vi "AutoSpotting.vi"(3 "spotfinding settings":T1={"show all"=FALSE, "threshold/morph"=FALSE, "particle filter"=FALSE, "spot marks"=FALSE, "close filter"=FALSE, "connectivity 4/8"=FALSE, "range"={"Lower value"=30.0, "Upper value"=30.0}, "PSF-size"=0, "Parameters"=[]} {"range"."Upper value" format="%.2f"; "range"."Lower value" format="%.2f"; "Parameters"."Upper Value" format="%.2f"; "Parameters"."Lower Value" format="%.2f"}, 4 "Intensity Image In":T2, 5 "already x spots":i16) -> (0 "coordinates":i32[][](array[numeric]), 1 "Number of Particles":i32)   [LabVIEW 2009]
uses:
  <vilib>/vision/Image Controls.llb/IMAQ Image.ctl
  spotfindersettings.ctl
  <vilib>/vision/NI_Vision_Development_Module.lvlib
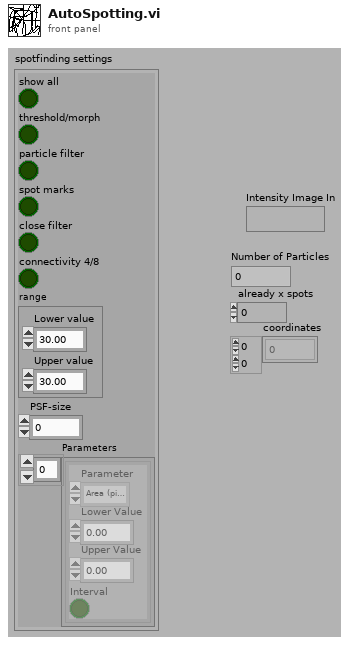
[diagram p1: front panel]
types:
  T1 = typedef "spotfindersettings.ctl" = cluster{"show all":bool, "threshold/morph":bool, "particle filter":bool, "spot marks":bool, "close filter":bool, "connectivity 4/8":bool, "range":cluster{"Lower value":sgl, "Upper value":sgl}, "PSF-size":i32, "Parameters":cluster{"Parameter":enum32{"Area (pixels)", "Area (calibrated)", "Number of holes", "Holes area (pixels)", "Total area (pixels)", "Scanned area (pixels)", "Ratio Area/Scanned area (%)", "Ratio Area/Total area (%)", "Center of mass (X)", "Center of mass (Y)", "Left column (X)", "Upper row (Y)", "Right column (X)", "Lower row (Y)", "Width (pixels)", "Height (pixels)", "Longest segment length", "Longest segment left column (X)", "Longest segment top row  (Y)", "Perimeter", "Holes perimeter", "SumX", "SumY", "SumXX", "SumYY", "SumXY", "Corrected projection X", "Corrected projection Y", "Moment of inertia Ixx", "Moment of inertia Iyy", "Moment of inertia Ixy", "Mean chord X", "Mean chord Y", "Max intercept", "Mean intercept perpendicular", "Particle orientation", "Equivalent ellipse minor axis", "Ellipse major axis", "Ellipse minor axis", "Ratio of equivalent ellipse axis", "Rectangle big side", "Rectangle small side", "Ratio of equivalent rectangle sides", "Elongation factor", "Compactness factor", "Heywood circularity factor", "Type factor", "Hydraulic radius", "Waddel disk diameter", "Diagonal"}, "Lower Value":sgl, "Upper Value":sgl, "Interval":bool}[]}
  T2 = typedef "IMAQ Image.ctl" = refnum<image>
  T3 = enum16{"Ini", "Get", "Set", "Refresh", "dump", "move", "name"}
  T4 = cluster{"Parameter":enum32{"Area (pixels)", "Area (calibrated)", "Number of holes", "Holes area (pixels)", "Total area (pixels)", "Scanned area (pixels)", "Ratio Area/Scanned area (%)", "Ratio Area/Total area (%)", "Center of mass (X)", "Center of mass (Y)", "Left column (X)", "Upper row (Y)", "Right column (X)", "Lower row (Y)", "Width (pixels)", "Height (pixels)", "Longest segment length", "Longest segment left column (X)", "Longest segment top row  (Y)", "Perimeter", "Holes perimeter", "SumX", "SumY", "SumXX", "SumYY", "SumXY", "Corrected projection X", "Corrected projection Y", "Moment of inertia Ixx", "Moment of inertia Iyy", "Moment of inertia Ixy", "Mean chord X", "Mean chord Y", "Max intercept", "Mean intercept perpendicular", "Particle orientation", "Equivalent ellipse minor axis", "Ellipse major axis", "Ellipse minor axis", "Ratio of equivalent ellipse axis", "Rectangle big side", "Rectangle small side", "Ratio of equivalent rectangle sides", "Elongation factor", "Compactness factor", "Heywood circularity factor", "Type factor", "Hydraulic radius", "Waddel disk diameter", "Diagonal"}, "Lower Value":sgl, "Upper Value":sgl, "Interval":bool}[]
  T5 = enum32{"AutoM", "Close", "Dilate", "Erode", "Gradient", "Gradient in", "Gradient out", "HitMiss", "Open", "PClose", "POpen", "Thick", "Thin"}
  T6 = cluster{"Area (pixels)":i32, "Area (calibrated)":sgl, "Perimeter":sgl, "Number of Holes":i32, "Hole's Area (pixels)":i32, "Hole's Perimeter":sgl, "Global Rectangle":cluster{"x1Left":i32, "y1Top":i32, "x2Right":i32, "y2Bottom":i32}, "åx":sgl, "åy":sgl, "åxx":sgl, " åyy":sgl, "åxy":sgl, "Longest Segment Length":i32, "Longest Segment Coordinates":cluster{"x":i32, "y":i32}, "Projection x":i32, "Projection y":i32}[]
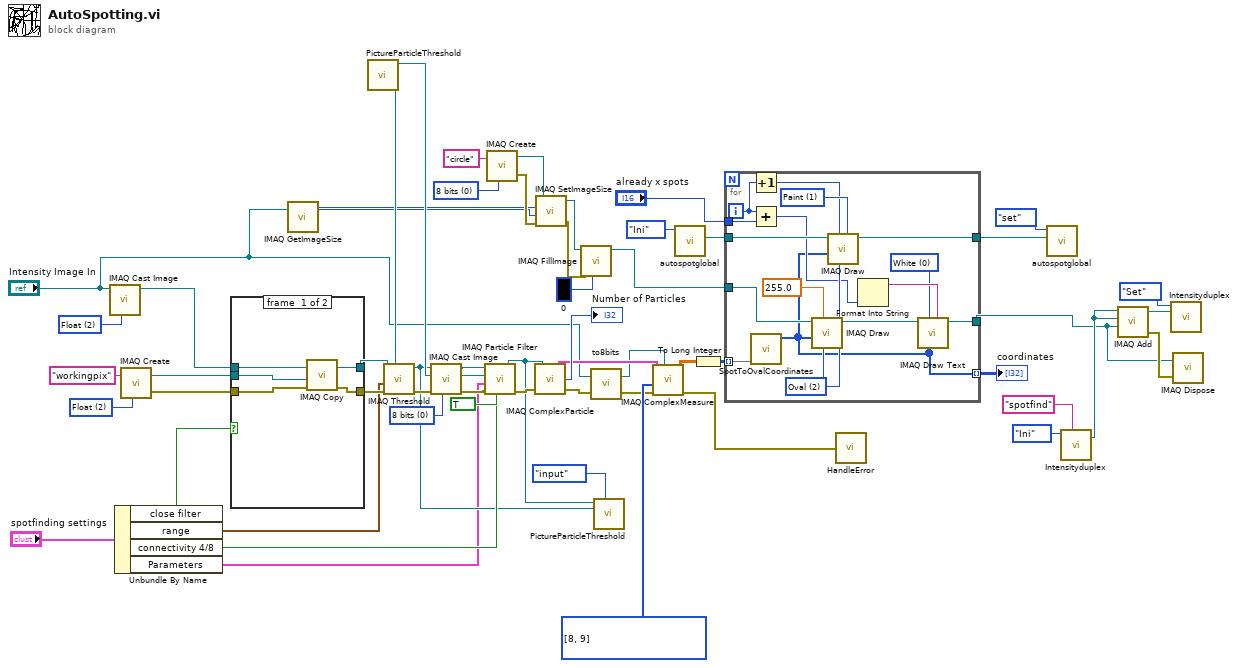
[diagram p0: block diagram]
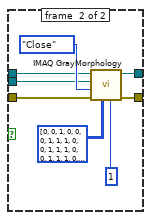
[diagram p2: hidden frame]
diagram:
  w20 = u32 0 items=["8 bits", "16 bits", "Float", "Complex", "RGB", "HSL"] ("Image Type")
  w36 = u32 0 items=["8 bits", "16 bits", "Float", "Complex", "RGB", "HSL"] ("Image Type")
  w40 = u32 2 items=["8 bits", "16 bits", "Float", "Complex", "RGB", "HSL"] ("Image Type")
  w52 = i32[] [8, 9] items=["Area (pixels)", "Area (calibrated)", "Number of holes", "Holes area (pixels)", "Total area", "Scanned area", "Ratio Area/Scanned area (%)", "Ratio Area/Total area (%)", "Center of mass (X)", "Center of mass (Y)", "Left column (X)", "Upper row (Y)", "Right column (X)", "Lower row (Y)", "Width", "Height", "Longest segment length", "Longest segment left column (X)", "Longest segment top row  (Y)", "Perimeter", "Hole's perimeter", "SumX", "SumY", "SumXX", "SumYY", "SumXY", "Corrected projection X", "Corrected projection Y", "Moment of inertia Ixx", "Moment of inertia Iyy", "Moment of inertia Ixy", "Mean chord X", "Mean chord Y", "Max intercept", "Mean intercept perpendicular", "Particle orientation", "Equivalent ellipse minor axis", "Ellipse major axis", "Ellipse minor axis", "Ratio of equivalent ellipse axis", "Rectangle big side", "Rectangle small side", "Ratio of equivalent rectangle sides", "Elongation factor", "Compactness factor", "Heywood circularity factor", "Type factor", "Hydraulic radius", "Waddel disk diameter", "Diagonal"] ("Parameters")
  w55 = u32 2 items=["8 bits", "16 bits", "Float", "Complex", "RGB", "HSL"] ("Image Type")
  n1 = call "IMAQ Cast Image"("Image Type"=w40, "Image Src"="Intensity Image In") -> ("Image Dst Out"=w41:T2)  [unwired: 8 in, 1 out]
  n2 = Unbundle By Name("spotfinding settings") -> ("close filter"=w28:bool, "range"=w2:cluster{"Lower value":sgl, "Upper value":sgl}, "connectivity 4/8"=w27:bool, "Parameters"=w6:T4)
  n3 = call "IMAQ Create"("Image Name"="workingpix", "Image Type"=w55) -> ("New Image"=w57:T2, "error out"=w56:errorcluster)  [unwired: 3 in]
  n4 = case shown="True" w28 {
    tunnel: w56 -> [w60 w68]
    tunnel: w41 -> [w62 w67]
    tunnel: [w61 w66] -> w34
    tunnel: [w59 w65] -> w39
    tunnel: w57 -> [w58 w64]
    frame #0 {
      n5 = call "IMAQ Copy"("error in (no error)"=w60, "Image Dst"=w58, "Image Src"=w62) -> ("error out"=w59:errorcluster, "Image Dst Out"=w61:T2)  [unwired: 3 in]
    }
    frame #1 {
      n6 = call "IMAQ GrayMorphology"("Number of iterations (1)"=1, "Structuring Element"=i32[][] [[0, 0, 1, 0, 0], [0, 1, 1, 1, 0], [0, 1, 1, 1, 0], [0, 1, 1, 1, 0], [0, 0, 1, 0, 0]], "error in (no error)"=w68, "Operation"=T5."Close", "Image Dst"=w64, "Image Src"=w67) -> ("error out"=w65:errorcluster, "Image Dst Out"=w66:T2)  [unwired: 4 in]
    }
  }
  n7 = call "IMAQ GetImageSize"("Image"="Intensity Image In") -> ("Y Resolution"=w11:i32, "X Resolution"=w12:i32)  [unwired: 3 in, 1 out]
  n8 = call "PictureParticleThreshold.vi"() -> ("Image Dst float"=w26:T2, "Image Dst 8bit"=w25:T2)  [unwired: 8 in]
  n9 = call "IMAQ Threshold"("error in (no error)"=w39, "Range"=w2, "Image Dst"=w26, "Image Src"=w34) -> ("error out"=w38:errorcluster, "Image Dst Out"=w24:T2)  [unwired: 6 in]
  n10 = call "IMAQ Cast Image"("Image Type"=w36, "error in (no error)"=w38, "Image Src"=w24) -> ("error out"=w37:errorcluster, "Image Dst Out"=w33:T2)  [unwired: 7 in]
  n11 = call "IMAQ Particle Filter"("Keep/Remove Particles"=TRUE, "Connectivity 4/8 (8)"=w27, "error in (no error)"=w37, "Selection Values"=w6, "Image Dst"=w25, "Image Src"=w33) -> ("error out"=w54:errorcluster, "Image Dst Out"=w23:T2)  [unwired: 2 in]
  n12 = call "IMAQ Create"("Image Name"="circle", "Image Type"=w20) -> ("New Image"=w10:T2, "error out"=w15:errorcluster)  [unwired: 3 in]
  n13 = call "IMAQ ComplexParticle"("error in (no error)"=w54, "Image"=w23) -> ("error out"=w32:errorcluster, "Number of Particles"=→"Number of Particles":i32, "Complex Reports"=w51:T6)  [unwired: 1 in]
  n14 = call "IMAQ SetImageSize"("error in (no error)"=w15, "Y Resolution"=w11, "X Resolution"=w12, "Image"=w10) -> ("error out"=w14:errorcluster, "Image Out"=w9:T2)  [unwired: 1 in]
  n15 = call "IMAQ FillImage"("Color Pixel Value"=u32 0, "error in (no error)"=w14, "Image"=w9) -> ("Image Out"=w7:T2)  [unwired: 7 in, 1 out]
  n16 = call "to8bits.vi"("error in (no error)"=w32, "Image"="Intensity Image In") -> ("error out"=w31:errorcluster, "Image"=w30:T2)
  n17 = call "PictureParticleThreshold.vi"("Enum"=enum16{"new", "input", "draw", "dump"}."input", "Image Input float"=w24, "Image Input 8bit"=w23) -> ()  [unwired: 5 in, 2 out]
  n18 = call "IMAQ ComplexMeasure"("Image"=w30, "error in (no error)"=w31, "Parameters"=w52, "Complex Reports"=w51) -> ("error out"=w1:errorcluster, "Coefficients (2D)"=w50:sgl[][])  [unwired: 4 in, 2 out]
  n19 = call "autospotglobal.vi"("Enum"=enum16{"Ini", "get", "dump", "set", "draw"}."Ini") -> ("New Image"=w45:T2)  [unwired: 6 in]
  n20 = To Long Integer(number=w50) -> (32bit integer=w3:i32[][])
  n21 = for {
    tunnel: w3 -> [w72] mode=indexing
    tunnel: w7 -> [w86]
    tunnel: w45 -> [w85]
    tunnel: [w83] -> w43
    tunnel: [w80] -> w16
    tunnel: "already x spots" -> [w78]
    tunnel: [w71] -> w4 mode=indexing
    i -> [w76]
    w74 = 0 items=["White", "Black", "Inverted", "Black on White", "White on Black"] ("Color")
    w79 = u16 2 items=["Line", "Rectangle", "Oval"] ("Shape to draw")
    w84 = u16 1 items=["Frame", "Paint", "Invert Frame", "Invert Paint"] ("Draw Mode")
    n22 = Increment(x=w76) -> (x+1=w75:i32)
    n23 = Add(x=w76, y=w78) -> (x+y=w77:i32)
    n24 = call "SpotToOvalCoordinates.vi"("Spot"=w72) -> ("oval coordinates"=w71:i32[])  [unwired: 4 in, 2 out]
    n25 = call "IMAQ Draw"("Shape to draw"=w79, "Pixel Color"=sgl 255.0, "Coordinates"=w71, "Image Src"=w86) -> ("Image Dst Out"=w82:T2)  [unwired: 6 in, 1 out]
    n26 = call "IMAQ Draw"("Draw Mode"=w84, "Shape to draw"=w79, "Pixel Color"=w75, "Coordinates"=w71, "Image Src"=w85) -> ("Image Dst Out"=w83:T2)  [unwired: 5 in, 1 out]
    n27 = Format Into String(w77) -> (resulting string=w81:string)  [unwired: 3 in, 1 out]
    n28 = call "IMAQ Draw Text"("String"=w81, "Insertion Point"=w71, "Color"=w74, "Image Src"=w82) -> ("Image Dst Out"=w80:T2)  [unwired: 4 in, 3 out]
  }
  "coordinates" <- w4
  n29 = call "HandleError.vi"("error in (no error)"=w1) -> ()
  n30 = call "autospotglobal.vi"("Image In"=w43, "Enum"=enum16{"Ini", "get", "dump", "set", "draw"}."set") -> ()  [unwired: 5 in, 1 out]
  n31 = call "Intensityduplex.vi"("Enum"=T3."Ini", "title"="spotfind") -> ("Image Duplicate (out)"=w18:T2)  [unwired: 3 in, 1 out]
  n32 = call "IMAQ Add"("Image Src A"=w18, "Image Dst"=w18, "Image Src B"=w16) -> ("Image Dst Out"=w19:T2, "error out"=w17:errorcluster)  [unwired: 4 in]
  n33 = call "Intensityduplex.vi"("Enum"=T3."Set", "Image In"=w19) -> ()  [unwired: 3 in, 2 out]
  n34 = call "IMAQ Dispose"("Image"=w16, "error in (no error)"=w17) -> ()  [unwired: 4 in, 1 out]
